vi "Binary to KLB(64-bit)Multiple Files.vi"() -> ()   [LabVIEW 2013]
uses:
  File IO/KLB/VIs/Type Defs/KLB Settings Cluster.ctl
  File IO/KLB/VIs/Type Defs/KLB # of CPUs enum.ctl
  File IO/KLB/VIs/Type Defs/KLB compression type enum.ctl
  <vilib>/vision/Image Controls.llb/IMAQ Image.ctl
  File IO/KLB/KLB.lvlib
panel:
  out "Processing File":i32
  in  "KLB Settings":T1={"Logical Cores"=enum."CPU 75%", "pixelSize (um)"=[1.0, 1.0, 1.0, 1.0, 1.0], "blockSize"=[96, 96, 8, 1, 1], "compressionType"=enum."BZip2", "metadata"=""} {"pixelSize (um)" min=0.01 max=10 step=0.01 format="%.2f"}
  out "Image":T4(plugin-control)
  out "KLB Conversion Time (ms)":u32=53091
  out "Image/Sector Size(bytes)":i64=3384359664
  in  "stop":bool
  out "Progress":u64(slide)=3579 max=5098 scale=0.0..4240.0
  out "Partial images in file?":bool
  out "# of Images":u32=3579
  out "error IO":errorcluster
  out "Height":u32=788
  out "Width":u32=1200
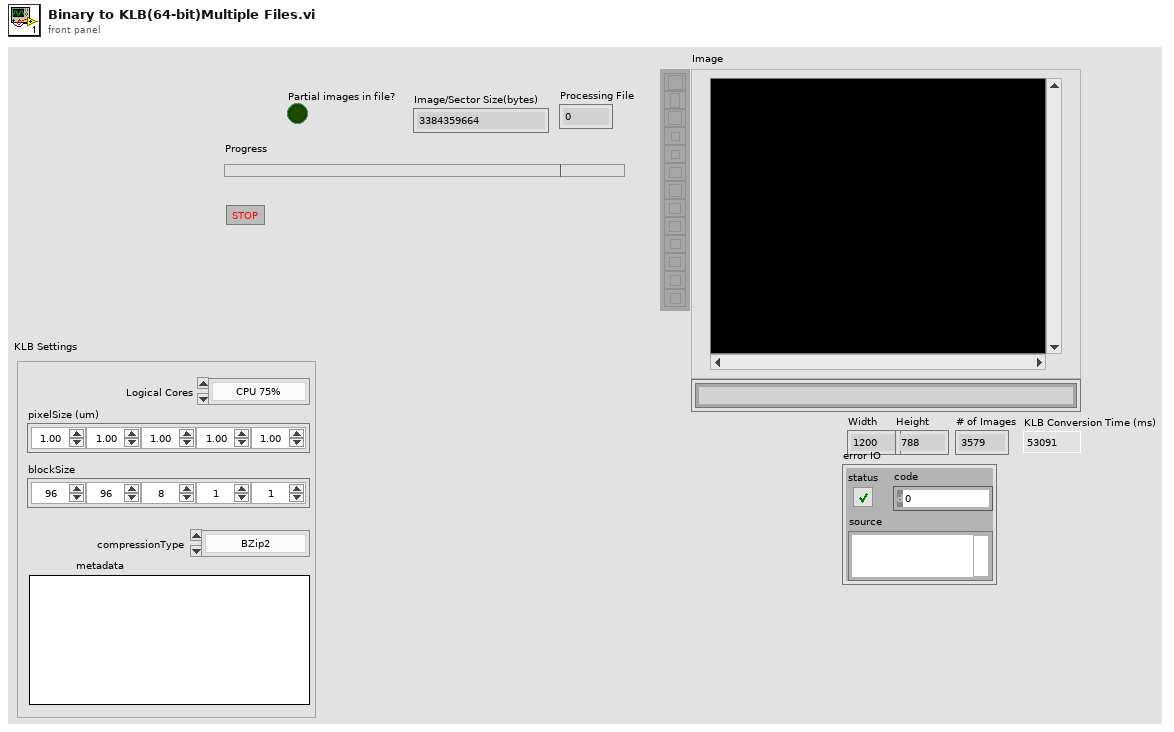
[diagram p1: front panel]
types:
  T1 = typedef "KLB.lvlib/KLB Settings Cluster.ctl" = cluster{"Logical Cores":T2, "pixelSize (um)":sgl[], "blockSize":u32[], "compressionType":T3, "metadata":string}
  T2 = typedef "KLB.lvlib/KLB # of CPUs enum.ctl" = enum16{"CPU 25%", "CPU 50%", "CPU 75%", "CPU All but 1", "1", "4", "8", "16"}
  T3 = typedef "KLB.lvlib/KLB compression type enum.ctl" = enum8{"Uncompressed", "BZip2"}
  T4 = typedef "IMAQ Image.ctl" = refnum<image>
  T5 = typedef "Mask ROI Cluster.ctl" = cluster{"left annulus":T6, "right annulus":T6, "Threshold Range":cluster{"Lower value":dbl, "Upper value":dbl}, "[Avg BG]":u8[], "Number of Sectors":u8, "Left ROI":T7, "Right ROI":T7, "Left Start Angle Duty Cycle":fxp<+,8,0>, "Left End Angle Duty Cycle":fxp<+,8,0>, "Right End Angle Duty Cycle":fxp<+,8,0>, "Right Start Angle Duty Cycle":fxp<+,8,0>, "[Sector ROIs]":T7[], "Consecutive Sector Threshold":u8}
  T6 = typedef "IMAQ Circle" = cluster{"Center X":i32, "Center Y":i32, "Inner Radius":i32, "Outer Radius":i32, "Start Angle":dbl, "End Angle":dbl}
  T7 = typedef "ROI Descriptor" = cluster{"Global Rectangle":i32[], "Contours":cluster{"ID":enum32{"External", "Internal"}, "Type":u32, "Coordinates":i32[]}[]}
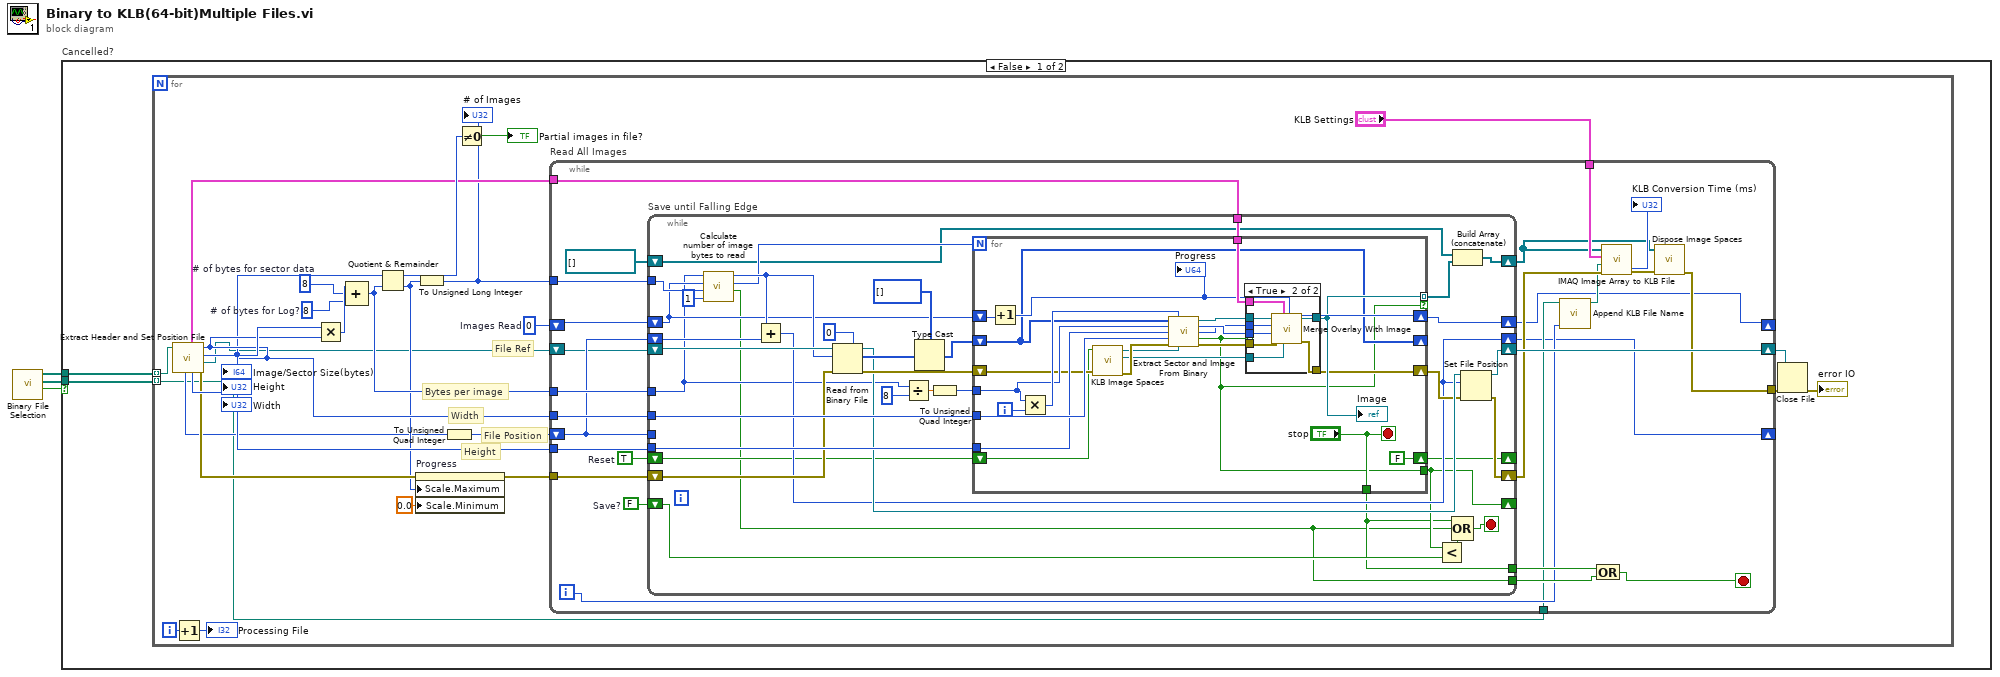
[diagram p0: block diagram]
diagram:
  n1 = call "Binary File Selection.vi"() -> ("cancelled"=w3:bool, "klb paths"=w1:path[], "selected paths"=w2:path[])  [unwired: 9 in]
  n2 = case "Cancelled?" shown="False" w3 {
    tunnel: w2 -> [w5 _]
    tunnel: w1 -> [w4 _]
    frame False {
      n3 = for {
        tunnel: w5 -> [w11] mode=indexing
        tunnel: w4 -> [w10] mode=indexing
        i -> [w7]
        w8 = u32 0  # Images Read
        w13 = u32 8  # # of bytes for Log?
        w26 = u32 8  # # of bytes for sector data
        # "File Position"
        # "Height"
        # "Width"
        # "Bytes per image"
        # "File Ref"
        n4 = call "Extract Header and Set Position File.vi"("Binary File"=w11) -> ("error out"=w21:errorcluster, "refnum out"=w16:refnum<file>, "Height"=w24:u32, "Width"=w23:u32, "Image/Sector Size(bytes)"=w22:i64, "Mask ROI Out"=w17:T5, "Header Size"=w19:i32)  [unwired: 4 in]
        "Width" <- w23
        "Height" <- w24
        "Image/Sector Size(bytes)" <- w22
        n5 = Increment(x=w7) -> (x+1=→"Processing File":i32)
        n6 = Multiply(x=w24, y=w23) -> (x*y=w27:u32)
        n7 = Compound Arithmetic op=ADD(w27, w26, w13) -> (w25:u32)
        n8 = Quotient & Remainder(x=w22, y=w25) -> (x-y*floor(x/y)=w31:i64, floor(x/y)=w20:i64)
        n9 = property on="Progress" class="Slide (strict)"(error in=w21, "Scale.Maximum"=w20, "Scale.Minimum"=0.0 ("Data Entry Limits:Minimum")) -> (error out=w29:errorcluster)  [unwired: 1 in, 1 out]
        n10 = To Unsigned Long Integer(number=w20) -> (unsigned 32bit integer=w15:u32)
        "# of Images" <- w15
        n11 = To Unsigned Quad Integer(1:w19) -> (0:w18:u64)
        n12 = Not Equal To 0?(x=w31) -> (x != 0?=→"Partial images in file?":bool)
        n13 = while "Read All Images" {
          tunnel: w29 -> [w58]
          tunnel: w25 -> [w57]
          tunnel: w24 -> [w56]
          tunnel: w23 -> [w55]
          tunnel: w17 -> [w53]
          tunnel: w15 -> [w51]
          tunnel: "KLB Settings" -> [w48]
          tunnel: w10 -> [w37]
          tunnel: [w43] -> w9
          shift-right: [w59] -> w30
          shift-left: w16 -> [w52]
          shift-right: [w34] -> _
          shift-left: w8 -> [w35]
          shift-right: [w33] -> _
          shift-left: w18 -> [w54]
          i -> [w38]
          stop <- w39 stop-if-true
          w42 = FALSE  # Save?
          w47 = TRUE  # Reset
          n14 = while "Save until Falling Edge" {
            tunnel: w55 -> [w96]
            tunnel: w56 -> [w95]
            shift-right: [w88] -> w44
            shift-left: w58 -> [w93]
            shift-right: [w86] -> w59
            shift-left: w52 -> [w94]
            tunnel: w57 -> [w74]
            tunnel: w54 -> [_]
            shift-right: [w78] -> w34
            shift-left: w35 -> [w79]
            tunnel: w51 -> [w85]
            shift-right: [w76] -> w33
            shift-left: w54 -> [w83]
            tunnel: w53 -> [w75]
            shift-right: [w68] -> w45
            shift-left: T4[] [] -> [w67]
            shift-right: [w65] -> _
            shift-left: w47 -> [w66]
            shift-right: [w64] -> _
            shift-left: w42 -> [w63]
            tunnel: [w61] -> w41
            tunnel: [w60] -> w40
            stop <- w84 stop-if-true
            n15 = call "Calculate number of image bytes to read.vi"("Images per Chunk"=u32 1, "# of total images"=w85, "Total Images Read"=w79, "# of bytes per image"=w74) -> ("All Images Read?"=w60:bool, "# of Images Read"=w80:u32, "# of bytes to read"=w82:u64)  [unwired: 5 in]
            n16 = Add(x=w82, y=w83) -> (x+y=w76:u64)
            n17 = Read from Binary File(5:u8 0, 8:w93, 10:w82, 11:w94) -> (0:w92:errorcluster, 2:w90:u8[], 3:w87:refnum<file>)  [unwired: 2 in, 1 out]
            n18 = Divide(x=w74, y=u32 8) -> (x/y=w72:dbl)
            n19 = Type Cast(type=u64[] [], x=w90) -> (*(type *) &x=w81:u64[])
            n20 = To Unsigned Quad Integer(1:w72) -> (0:w71:u64)
            n21 = for {
              N: w80 -> [_]
              tunnel: w96 -> [w117]
              tunnel: w95 -> [w116]
              shift-right: [w109] -> w78
              shift-left: w79 -> [w115]
              shift-right: [w106] -> w77
              shift-left: w92 -> [w103]
              tunnel: ["stop"] -> w61
              tunnel: w75 -> [w112]
              tunnel: w71 -> [w108]
              tunnel: [w107] -> w70 mode=indexing if=w97
              shift-right: [w104] -> _
              shift-left: w81 -> [w104]
              shift-right: [FALSE ("Reset")] -> w65
              shift-left: w66 -> [w99]
              tunnel: [w97] -> w64
              i -> [w119]
              stop <- "stop" stop-if-true
              n22 = Increment(x=w115) -> (x+1=w109:u32)
              "Progress" <- w109
              n23 = Multiply(x=w108, y=w119) -> (x*y=w118:u64)
              n24 = call "KLB Image Spaces.vi"("error in (no error)"=w103, "Reset?"=w99) -> ("error out"=w102:errorcluster, "RGB Image"=w100:T4, "U8 Image"=w101:T4)  [unwired: 7 in]
              n25 = call "Extract Sector and Image From Binary.vi"("Binary Data(u64)"=w104, "Start Index"=w118, "# of u64 per image"=w108, "Height"=w116, "Width"=w117, "error in (no error)"=w102, "Image Destination"=w101) -> ("Image Out"=w113:T4, "Left Sector"=w111:u16, "Right Sector"=w110:u16, "Log?"=w97:bool, "error out"=w105:errorcluster)  [unwired: 4 in]
              n26 = case shown="True" w97 {
                tunnel: w113 -> [w121 w129]
                tunnel: w112 -> [_ w128]
                tunnel: w111 -> [_ w127]
                tunnel: w110 -> [_ w126]
                tunnel: [w121 w125] -> w107
                tunnel: [w120 w124] -> w106
                tunnel: w105 -> [w120 w123]
                tunnel: w100 -> [_ w122]
                frame False {
                }
                frame True {
                  n27 = call "Merge Overlay With Image.vi"("Image RGB"=w122, "ROI Cluster"=w128, "Error in"=w123, "Left Edge"=w127, "Right Edge"=w126, "Image In"=w129) -> ("error out"=w124:errorcluster, "Image Out"=w125:T4)  [unwired: 4 in]
                }
              }
              "Image" <- w107
            }
            n28 = Less?(x=w64, y=w63) -> (x < y?=w62:bool)
            n29 = Compound Arithmetic op=OR(w61, w60, w62) -> (w84:bool)
            n30 = Build Array (concatenate)(w67, w70) -> (w68:T4[])
            n31 = Set File Position(offset (in bytes) (0)=w76, refnum=w87, error in=w77) -> (refnum out=w86:refnum<file>, error out=w88:errorcluster)  [unwired: 1 in]
          }
          n32 = call "Append KLB File Name.vi"("Iteration"=w38, "Path In"=w37) -> ("Path Out"=w36:path)  [unwired: 9 in]
          n33 = Compound Arithmetic op=OR(w41, w40) -> (w39:bool)
          n34 = call "IMAQ Image Array to KLB File.vi"("error in (no error)"=w44, "path"=w36, "KLB Settings"=w48, "Images to Compress"=w45) -> ("error out"=w46:errorcluster, "elapsed (ms)"=→"KLB Conversion Time (ms)":u32)  [unwired: 6 in]
          n35 = call "Dispose Image Spaces.vi"("error in (no error)"=w46, "[Images]"=w45) -> ("error out"=w43:errorcluster)  [unwired: 9 in]
        }
        n36 = Close File(refnum=w30, error in=w9) -> (error out=→"error IO":errorcluster)  [unwired: 1 out]
      }
    }
    frame True {
    }
  }
